vi "倒计时器.vi"() -> ()   [LabVIEW 2017]
panel:
  out "buling":bool
  out "倒计时":timestamp format="%<%M:%S>T"
  in  "开始":bool
  in  "停止":bool
  in  "定时时间选择":enum16{"6秒", "10秒", "20秒"}(ring)
  # "倒计时器"
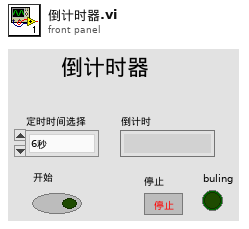
[diagram p1: front panel]
types:
  T1 = enum8{"Enabled", "Disabled", "Disabled and Grayed Out"}
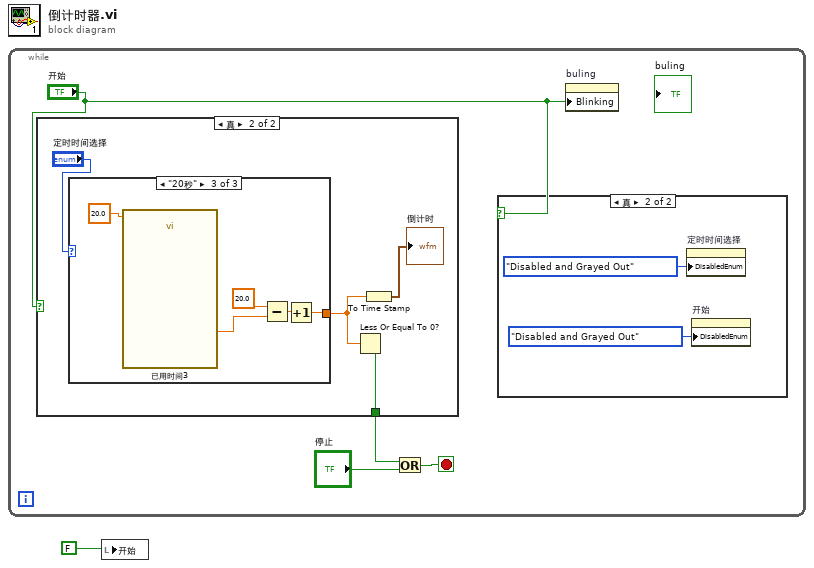
[diagram p0: block diagram]
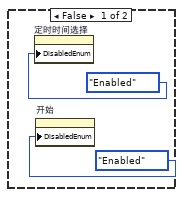
[diagram p2: hidden frame]
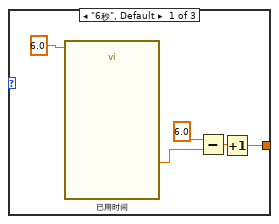
[diagram p4: hidden frame]
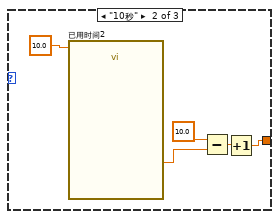
[diagram p5: hidden frame]
diagram:
  n1 = while {
    stop <- w3 stop-if-true
    n2 = case shown="真" "开始" {
      tunnel: [_ w11] -> w4
      frame False {
      }
      frame True {
        n3 = case shown="\"20秒\"" "定时时间选择" {
          tunnel: [w14 w19 w24] -> w12
          frame "6秒", Default {
            n4 = call "已用时间"("Time Target (s)"=6.0) -> ("Elapsed Time (s)"=w16:dbl)  [unwired: 11 in, 7 out]
            n5 = Subtract(x=6.0, y=w16) -> (x-y=w15:dbl)
            n6 = Increment(x=w15) -> (x+1=w14:dbl)
          }
          frame "10秒" {
            n7 = call "已用时间2"("Time Target (s)"=10.0) -> ("Elapsed Time (s)"=w21:dbl)  [unwired: 11 in, 7 out]
            n8 = Subtract(x=10.0, y=w21) -> (x-y=w20:dbl)
            n9 = Increment(x=w20) -> (x+1=w19:dbl)
          }
          frame "20秒" {
            n10 = call "已用时间3"("Time Target (s)"=20.0) -> ("Elapsed Time (s)"=w26:dbl)  [unwired: 11 in, 7 out]
            n11 = Subtract(x=20.0, y=w26) -> (x-y=w25:dbl)
            n12 = Increment(x=w25) -> (x+1=w24:dbl)
          }
        }
        n13 = Less Or Equal To 0?(x=w12) -> (x <= 0?=w11:bool)
        n14 = To Time Stamp(1:w12) -> (0:→"倒计时":timestamp)
      }
    }
    n15 = Or(x=w4, y="停止") -> (x .or. y?=w3:bool)
    n16 = case shown="真" "开始" {
      frame False {
        n17 = property on="定时时间选择" class="Enum (严格)"("DisabledEnum"=T1."Enabled" ("禁用")) -> ()  [unwired: 2 in, 2 out]
        n18 = property on="开始" class="Bool (严格)"("DisabledEnum"=T1."Enabled" ("禁用")) -> ()  [unwired: 2 in, 2 out]
      }
      frame True {
        n19 = property on="定时时间选择" class="Enum (严格)"("DisabledEnum"=T1."Disabled and Grayed Out" ("禁用")) -> ()  [unwired: 2 in, 2 out]
        n20 = property on="开始" class="Bool (严格)"("DisabledEnum"=T1."Disabled and Grayed Out" ("禁用")) -> ()  [unwired: 2 in, 2 out]
      }
    }
    n21 = property on="buling" class="Bool (严格)"("Blinking"="开始") -> ()  [unwired: 2 in, 2 out]
  }
  n22 = local write "开始"(FALSE) -> ()
